vi "Get Process State.vi"(5 "Publish State? (T)":bool=TRUE, 8 "error in (no error)":errorcluster, 11 "Process in":refnum<class "Process.lvclass">) -> (0 "error out":errorcluster, 1 "Payload":variant, 2 "Command":string, 3 "Process out":refnum<class "Process.lvclass">)   [LabVIEW 2019, in "TimingDRV Engine.lvlib" / "Process.lvclass"]
uses:
  Process.lvclass
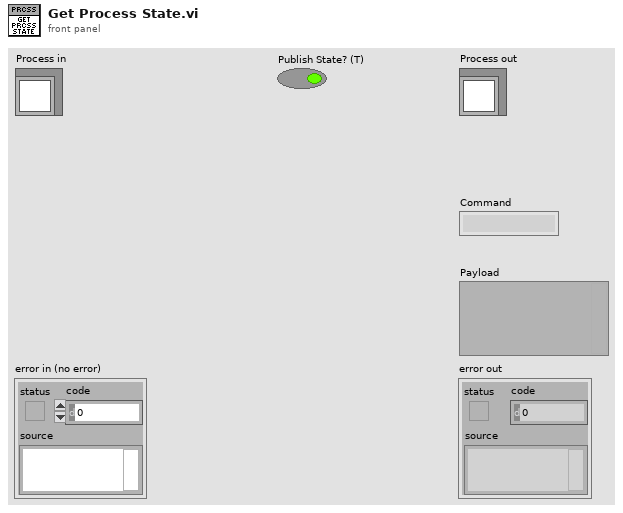
[diagram p1: front panel]
types:
  T1 = typedef "TimingDRV Engine.lvlib/Process.lvclass/Process Lookup.ctl" = cluster{"Process ID":string, "MessageQ":refnum<queue>, "Update UE":refnum<user-event>}
  T2 = typedef "TimingDRV Engine.lvlib/Process.lvclass/Message.ctl" = cluster{"Command":string, "Payload":variant}
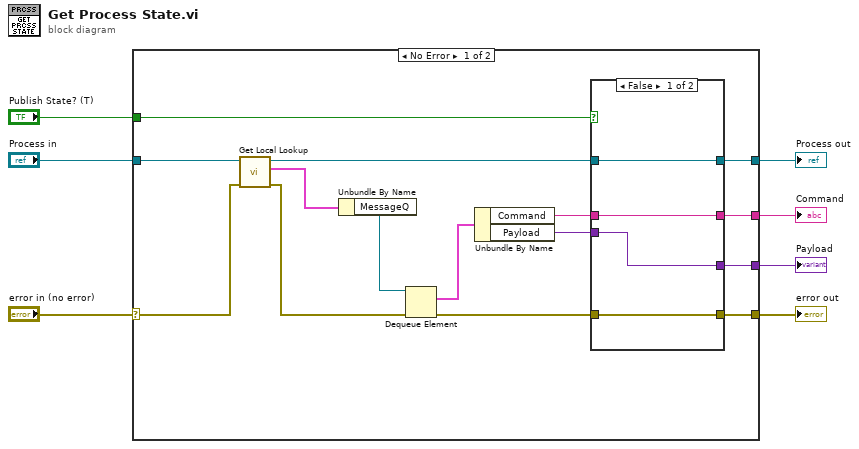
[diagram p0: block diagram]
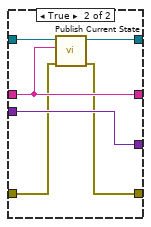
[diagram p2: hidden frame]
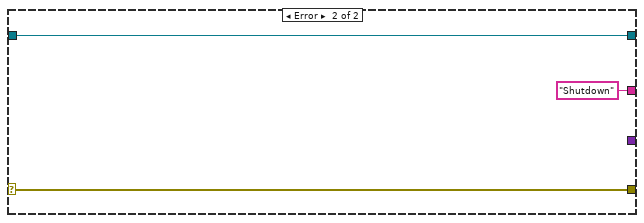
[diagram p3: hidden frame]
diagram:
  n1 = case shown="No Error" "error in (no error)" {
    selector: "error in (no error)" -> [w18 w35]
    tunnel: [w8 w35] -> w6
    tunnel: [w15 w34] -> w4
    tunnel: "Process in" -> [w19 w34]
    tunnel: [w10 _] -> w3
    tunnel: "Publish State? (T)" -> [w13 _]
    tunnel: [w11 "Shutdown" ("Command")] -> w1
    frame No Error {
      n2 = call-dynamic "Get Local Lookup.vi"("error in (no error)"=w18, "Process in"=w19) -> ("error out"=w17:errorcluster, "Process Lookup"=w22:T1, "Process out"=w16:refnum<class "Process.lvclass">)  [unwired: 7 in]
      n3 = Unbundle By Name(w22) -> ("MessageQ"=w21:refnum<queue>)
      n4 = Dequeue Element(queue=w21, error in (no error)=w17) -> (element=w20:T2, error out=w9:errorcluster)  [unwired: 1 in, 2 out]
      n5 = Unbundle By Name(w20) -> ("Command"=w14:string, "Payload"=w12:variant)
      n6 = case shown="False" w13 {
        tunnel: w16 -> [w24 w32]
        tunnel: [w24 w31] -> w15
        tunnel: w14 -> [w26 w29]
        tunnel: w12 -> [w25 w30]
        tunnel: [w25 w30] -> w10
        tunnel: [w26 w29] -> w11
        tunnel: w9 -> [w23 w28]
        tunnel: [w23 w27] -> w8
        frame False {
        }
        frame True {
          n7 = call "Publish Current State.vi"("error in (no error)"=w28, "State"=w29, "Process in"=w32) -> ("error out"=w27:errorcluster, "Process out"=w31:refnum<class "Process.lvclass">)  [unwired: 7 in]
        }
      }
    }
    frame Error {
    }
  }
  "error out" <- w6
  "Process out" <- w4
  "Command" <- w1
  "Payload" <- w3
